vi "Detect_Particle-8.vi"(4 "[IN] Filtering Settings":T1, 5 "Keep Nega-\ntive Values?":bool, 6 "# Channel":u8, 7 "Particle Searching Settings":T4 {"Type of particle filter"."Measurement Parameter" items=["Center of Mass X", "Center of Mass Y", "First Pixel X", "First Pixel Y", "Bounding Rect Left", "Bounding Rect Top", "Bounding Rect Right", "Bounding Rect Bottom", "Max Feret Diameter Start X", "Max Feret Diameter Start Y", "Max Feret Diameter End X", "Max Feret Diameter End Y", "Max Horiz. Segment Length Left", "Max Horiz. Segment Length Right", "Max Horiz. Segment Length Row", "-", "Bounding Rect Width", "Bounding Rect Height", "Bounding Rect Diagonal", "Perimeter", "Convex Hull Perimeter", "Holes' Perimeter", "Max Feret Diameter", "Equivalent Ellipse Major Axis", "Equivalent Ellipse Minor Axis", "Equivalent Ellipse Minor Axis (Feret)", "Equivalent Rect Long Side", "Equivalent Rect Short Side", "Equivalent Rect Diagonal", "Equivalent Rect Short Side (Feret)", "Average Horiz. Segment Length", "Average Vert. Segment Length", "Hydraulic Radius", "Waddel Disk Diameter", "-", "Area", "Holes' Area", "Particle & Holes' Area", "Convex Hull Area", "Image Area", "-", "Number of Holes", "Number of Horiz. Segments", "Number of Vert. Segments", "-", "Orientation", "Max Feret Diameter Orientation", "-", "% Area/Image Area", "% Area/(Particle & Holes' Area)", "Ratio of Equivalent Ellipse Axes", "Ratio of Equivalent Rect Sides", "-", "Elongation Factor", "Compactness Factor", "Heywood Circularity Factor", "Type Factor", "-", "Sum X", "Sum Y", "Sum XX", "Sum XY", "Sum YY", "Sum XXX", "Sum XXY", "Sum XYY", "Sum YYY", "-", "Moment of Inertia XX", "Moment of Inertia XY", "Moment of Inertia YY", "Moment of Inertia XXX", "Moment of Inertia XXY", "Moment of Inertia XYY", "Moment of Inertia YYY", "Norm. Moment of Inertia XX", "Norm. Moment of Inertia XY", "Norm. Moment of Inertia YY", "Norm. Moment of Inertia XXX", "Norm. Moment of Inertia XXY", "Norm. Moment of Inertia XYY", "Norm. Moment of Inertia YYY", "Hu Moment 1", "Hu Moment 2", "Hu Moment 3", "Hu Moment 4", "Hu Moment 5", "Hu Moment 6", "Hu Moment 7"]}, 8 "error IN":errorcluster, 9 "Binarization Settings":cluster{"MinBin2":sgl, "MaxBin2":sgl}[](array[cluster]), 10 "[IN] Destination Image":T2, 11 "[IN] Frame":T2) -> (0 "error OUT":errorcluster, 2 "[OUT] Particle Reports (Pixels)":T5(array[cluster]) {"Orientation" format="%.2f"; "Dimensions"."Height" format="%.2f"; "Dimensions"."Width" format="%.2f"; "Center of Mass"."Y" format="%.2f"; "Center of Mass"."X" format="%.2f"; "Bounding Rect"."Bottom" format="%.2f"; "Bounding Rect"."Right" format="%.2f"; "Bounding Rect"."Top" format="%.2f"; "Bounding Rect"."Left" format="%.2f"; "Number of Holes" format="%.2f"; "Area" format="%.2f"}, 3 "[OUT] Binarized Image":T2)   [LabVIEW 2013]
doc: "SubVI demonstrates the resulting localization of particles with selected parameters"
uses:
  <vilib>/vision/Image Controls.llb/IMAQ Image.ctl
  <vilib>/vision/NI_Vision_Development_Module.lvlib
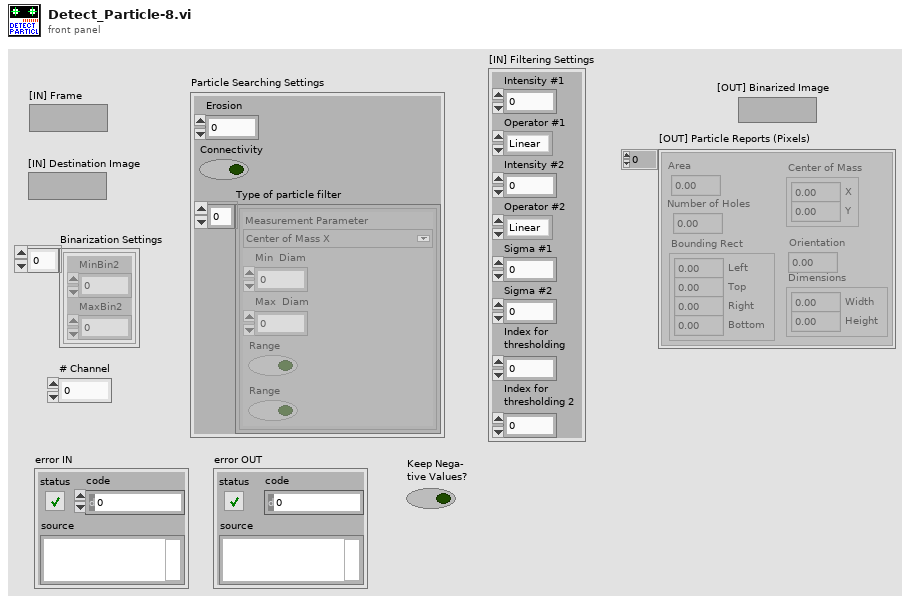
[diagram p1: front panel]
types:
  T1 = cluster{"Intensity #1":sgl, "Operator #1":enum32{"Linear", "Log", "Exp", "Square", "Square root", "Power X", "Power 1/X"}, "Intensity #2":sgl, "Operator #2":enum32{"Linear", "Log", "Exp", "Square", "Square root", "Power X", "Power 1/X"}, "Sigma #1":dbl, "Sigma #2":dbl, "Index for \nthresholding":u8, "Index for \nthresholding 2":u8}
  T2 = typedef "IMAQ Image.ctl" = refnum<image>
  T3 = typedef "Particle Parameters" = i32
  T4 = cluster{"Erosion":i32, "Connectivity ":bool, "Type of particle filter":cluster{"Measurement Parameter":T3, "Min  Diam":dbl, "Max  Diam":dbl, "Range":bool, "Range":bool}[]}
  T5 = cluster{"Area":dbl, "Number of Holes":dbl, "Bounding Rect":cluster{"Left":dbl, "Top":dbl, "Right":dbl, "Bottom":dbl}, "Center of Mass":cluster{"X":dbl, "Y":dbl}, "Orientation":dbl, "Dimensions":cluster{"Width":dbl, "Height":dbl}}[]
  T6 = enum32{"Linear", "Log", "Exp", "Square", "Square root", "Power X", "Power 1/X"}
  T7 = cluster{"Starting Value":sgl, "Incremental Value":sgl, "Histogram":u32[]}
  T8 = cluster{"Measurement Parameter":T3, "Min  Diam":dbl, "Max  Diam":dbl, "Range":bool, "Range":bool}[]
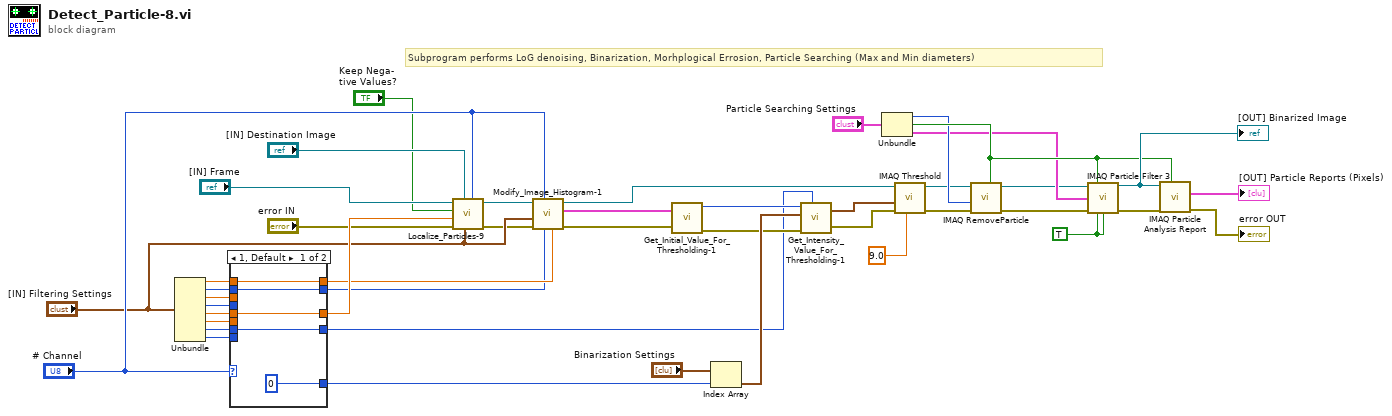
[diagram p0: block diagram]
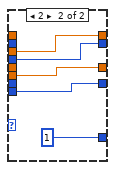
[diagram p2: hidden frame]
diagram:
  w44 = TRUE ("Fill Holes? (F)")
  # "Subprogram performs LoG denoising, Binarization, Morhplogical Errosion, Particle Searching (Max and Min diameters)"
  n1 = Unbundle("[IN] Filtering Settings") -> ("Intensity #1"=w10:sgl, "Operator #1"=w9:T6, "Intensity #2"=w6:sgl, "Operator #2"=w5:T6, "Sigma #1"=w34:dbl, "Sigma #2"=w33:dbl, "Index for \nthresholding"=w32:u8, "Index for \nthresholding 2"=w31:u8)
  n2 = case shown="1, Default" "# Channel" {
    tunnel: w34 -> [w48 _]
    tunnel: w33 -> [_ w53]
    tunnel: w32 -> [w47 _]
    tunnel: w31 -> [_ w52]
    tunnel: [0 1] -> w29
    tunnel: [w48 w53] -> w16
    tunnel: [w47 w52] -> w19
    tunnel: [w46 w51] -> w8
    tunnel: w10 -> [w46 _]
    tunnel: [w45 w50] -> w7
    tunnel: w9 -> [w45 _]
    tunnel: w6 -> [_ w51]
    tunnel: w5 -> [_ w50]
    frame 1, Default {
    }
    frame 2 {
    }
  }
  n3 = call "Localize_Particles-9.vi"("# channel"="# Channel", "[IN] Filtering Settings"="[IN] Filtering Settings", "[IN] Destination Image"="[IN] Destination Image", "error IN"="error IN", "[IN] Sigma"=w16, "Keep Nega-\ntive Values?"="Keep Nega-\ntive Values?", "[IN] Frame"="[IN] Frame") -> ("error OUT"=w11:errorcluster, "[OUT] LoG Processed Image"=w14:T2)  [unwired: 1 in, 1 out]
  n4 = call "Modify_Image_Histogram-1.vi"("[IN] Parameter"=w8, "[IN] Operator"=w7, "# channel"="# Channel", "error IN"=w11, "[IN] Filtering Settings"="[IN] Filtering Settings", "[IN] LoG Processed Image"=w14) -> ("error OUT"=w2:errorcluster, "[OUT] Histogram"=w3:T7, "[OUT] Histogram Modified Image"=w4:T2)  [unwired: 2 in, 1 out]
  n5 = call "Get_Initial_Value_For_Thresholding-1.vi"("[IN] Histogram Graph"=w3, "error IN"=w2) -> ("[OUT] Index of starting \npoint for thresholding"=w28:i32, "error OUT"=w26:errorcluster)  [unwired: 2 out]
  n6 = Index Array(array="Binarization Settings", index=w29) -> (element=w27:cluster{"MinBin2":sgl, "MaxBin2":sgl})
  n7 = call "Get_Intensity_Value_For_Thresholding-1.vi"("[IN] Index of starting \npoint for thresholding"=w28, "[IN] Thresholding range"=w27, "error IN"=w26, "[IN] Index for \nthresholding"=w19) -> ("[OUT] Thresholding range"=w25:cluster{"Lower value":sgl, "Upper value":sgl}, "error OUT"=w24:errorcluster)  [unwired: 1 in]
  n8 = Unbundle("Particle Searching Settings") -> ("Erosion"=w38:i32, "Connectivity"=w39:bool, "Type of particle filter"=w37:T8)
  n9 = call "IMAQ Threshold"("Replace Value"=sgl 9.0, "error in (no error)"=w24, "Range"=w25, "Image Src"=w4) -> ("error out"=w23:errorcluster, "Image Dst Out"=w22:T2)  [unwired: 6 in]
  n10 = call "IMAQ RemoveParticle"("Connectivity 4/8 (8)"=w39, "error in (no error)"=w23, "Number of Erosion"=w38, "Image Src"=w22) -> ("error out"=w35:errorcluster, "Image Dst Out"=w36:T2)  [unwired: 6 in]
  n11 = call "IMAQ Particle Filter 3"("Image Src"=w36, "Connectivity 4/8 (8)"=w39, "Selection Values"=w37, "error in (no error)"=w35, "Reject Border? (F)"=w44, "Fill Holes? (F)"=w44) -> ("Image Dst Out"=w43:T2, "error out"=w42:errorcluster)  [unwired: 7 in, 1 out]
  "[OUT] Binarized Image" <- w43
  n12 = call "IMAQ Particle Analysis Report"("Connectivity 4/8 (8)"=w39, "error in (no error)"=w42, "Image"=w43) -> ("error out"=→"error OUT":errorcluster, "Particle Reports (Pixels)"=→"[OUT] Particle Reports (Pixels)":T5)  [unwired: 3 in, 4 out]
